vi "Y to D Conversion.vi"   [LabVIEW 2014, in "NI_EP_Power Quality.lvlib"]
doc: "Converts phase voltages to line voltages. You must manually select the polymorphic instance you want to use.\n\nThis VI supports measuring single-line and multiple-line systems."
uses:
  <vilib>/addons/Electrical Power/PQ/NI_EP_Power Quality.lvlib
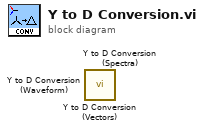
[diagram p0: block diagram]
diagram:
  n1 = call <vilib>:"Y to D Conversion (Vectors).vi"() -> ()  [unwired: 13 in, 3 out]
  n2 = call <vilib>:"Y to D Conversion (Spectra).vi"() -> ()  [unwired: 13 in, 3 out]
  n3 = call <vilib>:"Y to D Conversion (Waveform).vi"() -> ()  [unwired: 13 in, 3 out]
